vi "Continuous Measurament RT.vi"() -> ()   [LabVIEW 2014]
uses:
  <vilib>/FPGAPlugInAG/sbRIO-9636/niLvFpga_Open_sbRIO-9636.vi
  <vilib>/rvi/interface/common/dynamic/niFpgaDynamicAddResources.vi
  <vilib>/FPGAPlugInAG/Dynamic/niLvFpga_Reset_Dynamic.vi
  <vilib>/FPGAPlugInAG/Dynamic/niLvFpga_Run_Dynamic.vi
  <vilib>/FPGAPlugInAG/Dynamic/niLvFpga_Abort_Dynamic.vi
  <vilib>/FPGAPlugInAG/Dynamic/niLvFpga_Close_Dynamic.vi
  <vilib>/rvi/interface/nirviOpenFPGA/nirviOpenFPGA.xnode
  FPGA Bitfiles/FinalProjectLase_FPGATarget_ContinuousMeasur_qAypivenTJk.lvbitx
  FPGA/Continuous Measurement.vi
  <vilib>/rvi/interface/nirviMethod/nirviMethod.xnode
  <vilib>/rvi/interface/nirviCloseFPGA/nirviCloseFPGA.xnode
  <vilib>/Analysis/NI_AALBase.lvlib
panel:
  in  "Tab Control":T1(tab)
  in  "#Signals":u32(slide)=5 scale=1.0..5.0
  in  "Uncompensated":bool
  in  "Enable triangular scaling":bool=TRUE
  in  "Multiply Factor":dbl[](array[numeric])=[1.0, 0.8, 0.95, 0.85, 0.9]
  in  "Window function":enum16{"None", "Hanning"}(ring)=enum."Hanning"
  in  "Initial Latency points":u32(slide)=260 scale=0.0..1250.0
  in  "lower limit 1":u32(slide)=113 scale=0.0..113.0
  in  "lower limit 2":u32(slide)=738 scale=625.0..738.0
  in  "First FFT bin":i32=5
  in  "Last FFT bin":i32=255
  in  "Extraction Type":T2(ring)=enum."LowPass"
  in  "Low cutoff frequency":dbl=1000000.0 format="%#_13g"
  in  "Poly Grade":dbl=5.0
  in  "side points":i32=6
  in  "polynomial order":i32=3
  out "Distance (m)":dbl format="%0.7f"
  out "Relative Standard Deviation":dbl format="%0.7f"
  in  "Mean distance":i32=1
  out "Measure cycle time":u32
  out "Measurement Uncertainty (m)":dbl format="%0.5f"
  out "Measure Frequency":dbl
  out "Distance (m) Plot":dbl(graph)
  out "Velocity (m/s)":dbl
  out "Velocity (m/s) Plot":dbl(graph)
  in  "STOP":bool
  # "Modulation signal"
  # "Window function"
  # "Residual Extraction"
  # "FFT Parameters"
  # "Low pass filter"
  # "Compensated"
  # "Poly fitting"
  # "SavGolay filter"
  # "Performance"
  # "KHz"
  # "ms"
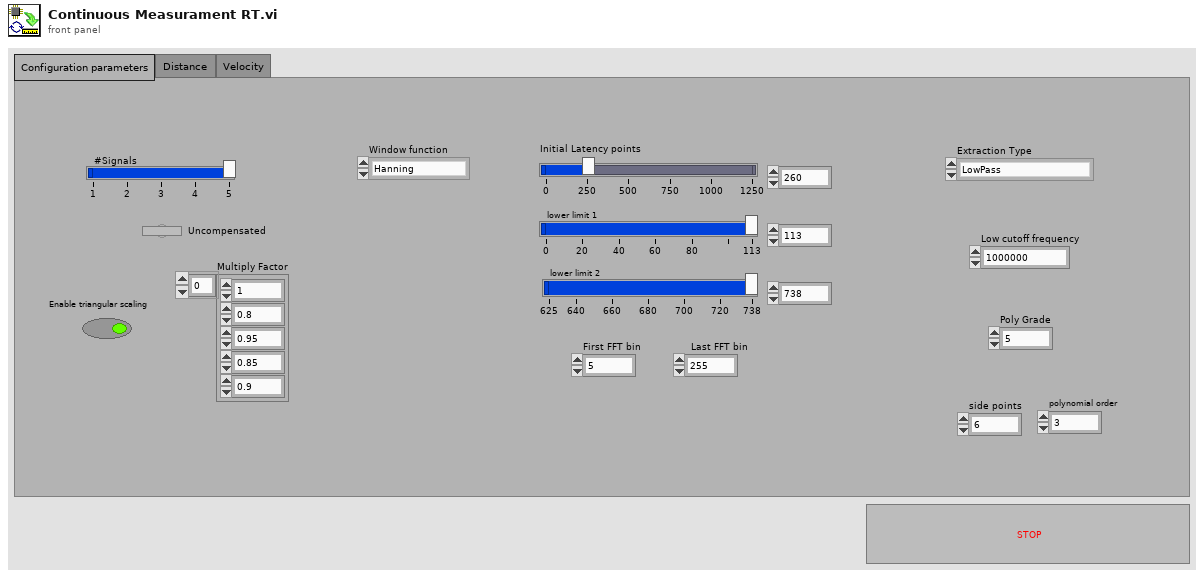
[diagram p1: front panel]
types:
  T1 = enum32{"Configuration parameters", "Distance ", "Velocity"}
  T2 = enum16{"NoSubtract", "StartingCurve", "LowPass", "PolyFitting", "SavGolay"}
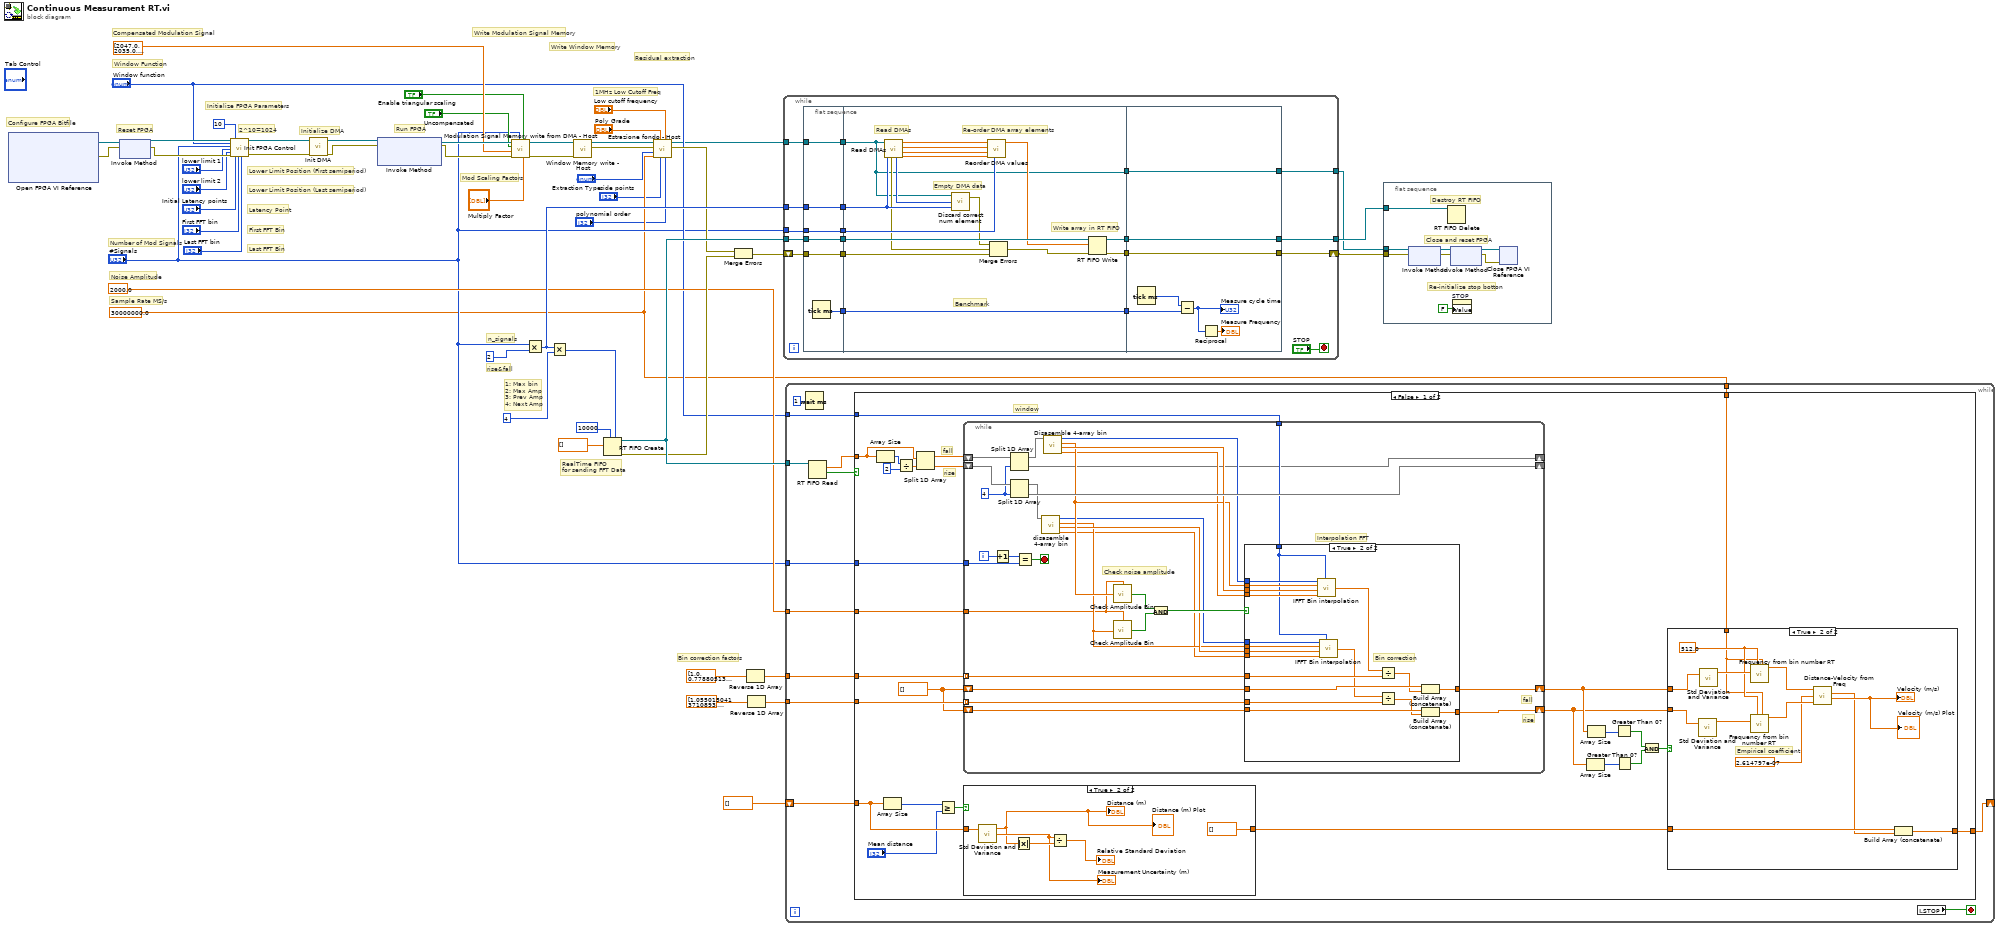
[diagram p0: block diagram]
diagram:
  w10 = 30000000.0
  # "2^10=1024"
  # "Bin correction factors"
  # "Write Modulation Signal Memory"
  # "Residual extraction"
  # "Write Window Memory"
  # "Mod Scaling Factors"
  # "Window Function"
  # "Lower Limit Position (Last semiperiod)"
  # "Lower Limit Position (First semiperiod)"
  # "Latency Point"
  # "Last FFT Bin"
  # "First FFT Bin"
  # "Number of Mod Signals"
  # "Configure FPGA Bitfile"
  # "Run FPGA"
  # "Reset FPGA"
  # "Initialize FPGA Parameters"
  # "Initialize DMA"
  # "1MHz Low Cutoff Freq"
  # "Compensated Modulation Signal"
  # "Sample Rate MS/s"
  # "Noise Amplitude"
  # "n_signals"
  # "rise&fall"
  # "1: Max bin\n2: Max Amp\n3: Prev Amp\n4: Next Amp"
  # "RealTime FIFO \nfor sending FFT Data"
  n1 = xnode "Open FPGA VI Reference"() -> ("FPGA VI Reference Out"=w21:refnum<k20>, "error out"=w20:errorcluster)  [unwired: 2 in]
  n2 = xnode "Invoke Method"("FPGA VI Reference In"=w21, "error in"=w20) -> ("FPGA VI Reference Out"=w18:refnum<k20>, "error out"=w19:errorcluster)
  n3 = call "Init FPGA Control.vi"("FPGA VI Reference In"=w18, "Window Function"="Window function", "n"="#Signals", "lower limit 1"="lower limit 1", "lower limit 2"="lower limit 2", "error in"=w19, "n-bit (2^(nbit) signals for Residual Extraction)"=10, "Initial Latency points"="Initial Latency points", "first FFT bin"="First FFT bin", "last FFT bin"="Last FFT bin") -> ("FPGA VI Reference Out"=w23:refnum<k20>, "error out"=w22:errorcluster)  [unwired: 8 in]
  n4 = call "Init DMA.vi"("error in"=w22, "FPGA VI Reference In"=w23) -> ("error out"=w24:errorcluster, "FPGA VI Reference Out"=w25:refnum<k20>)  [unwired: 8 in]
  n5 = xnode "Invoke Method"("FPGA VI Reference In"=w25, "error in"=w24) -> ("FPGA VI Reference Out"=w38:refnum<k20>, "error out"=w34:errorcluster)  [unwired: 1 in]
  n6 = call "Modulation Signal Memory write from DMA - Host.vi"("Triangular Multiply Factor"="Multiply Factor", "Enable triangular scaling"="Enable triangular scaling", "n"="#Signals", "error in"=w34, "Custom Triangular Signal (fal-ris)"=dbl[] [2047.0, 2035.0, 2022.0, 2010.0, 1997.0, 1985.0, 1972.0, 1960.0, 1948.0, 1935.0, 1923.0, 1911.0, 1899.0, 1886.0, 1874.0, 1862.0, 1850.0, 1838.0, 1825.0, 1813.0, 1801.0, 1789.0, 1777.0, 1765.0, 1753.0, 1741.0, 1729.0, 1717.0, 1705.0, 1693.0, 1681.0, 1669.0, 1657.0, 1645.0, 1634.0, 1622.0, 1610.0, 1598.0, 1586.0, 1575.0, 1563.0, 1551.0, 1540.0, 1528.0, 1516.0, 1505.0, 1493.0, 1481.0, 1470.0, 1458.0, 1447.0, 1435.0, 1424.0, 1412.0, 1401.0, 1389.0, 1378.0, 1366.0, 1355.0, 1344.0, 1332.0, 1321.0, 1310.0, 1298.0, 1287.0, 1276.0, 1265.0, 1253.0, 1242.0, 1231.0, 1220.0, 1209.0, 1198.0, 1186.0, 1175.0, 1164.0, 1153.0, 1142.0, 1131.0, 1120.0, 1109.0, 1098.0, 1087.0, 1076.0, 1065.0, 1055.0, 1044.0, 1033.0, 1022.0, 1011.0, 1000.0, 990.0, 979.0, 968.0, 958.0, 947.0, 936.0, 926.0, 915.0, 904.0, 894.0, 883.0, 873.0, 862.0, 852.0, 841.0, 831.0, 820.0, 810.0, 799.0, 789.0, 778.0, 768.0, 758.0, 747.0, 738.0, 727.0, 719.0, 712.0, 706.0, 700.0, 693.0, 687.0, 680.0, 674.0, 668.0, 661.0, 655.0, 648.0, 642.0, 636.0, 629.0, 623.0, 617.0, 610.0, 604.0, 598.0, 591.0, 584.0, 577.0, 569.0, 560.0, 552.0, 545.0, 538.0, 531.0, 525.0, 519.0, 512.0, 506.0, 500.0, 494.0, 488.0, 482.0, 476.0, 470.0, 464.0, 458.0, 452.0, 446.0, 436.0, 430.0, 424.0, 418.0, 412.0, 406.0, 400.0, 394.0, 388.0, 382.0, 376.0, 370.0, 364.0, 358.0, 352.0, 346.0, 338.0, 332.0, 325.0, 319.0, 313.0, 307.0, 301.0, 295.0, 290.0, 284.0, 278.0, 272.0, 267.0, 261.0, 255.0, 249.0, 244.0, 238.0, 232.0, 227.0, 221.0, 215.0, 209.0, 204.0, 198.0, 192.0, 187.0, 181.0, 175.0, 170.0, 164.0, 158.0, 153.0, 147.0, 141.0, 136.0, 130.0, 124.0, 119.0, 113.0, 108.0, 102.0, 96.0, 91.0, 85.0, 79.0, 74.0, 68.0, 62.0, 57.0, 51.0, 45.0, 39.0, 34.0, 28.0, 22.0, 16.0, 11.0, 5.0, 0.0, -6.0, -11.0, -17.0, -22.0, -28.0, -33.0, -39.0, -44.0, -50.0, -55.0, -61.0, -66.0, -72.0, -77.0, -83.0, -88.0, -94.0, -99.0, -105.0, -110.0, -116.0, -121.0, -127.0, -132.0, -137.0, -143.0, -148.0, -154.0, -159.0, -165.0, -170.0, -176.0, -181.0, -186.0, -192.0, -197.0, -203.0, -208.0, -214.0, -219.0, -224.0, -230.0, -235.0, -241.0, -246.0, -251.0, -257.0, -262.0, -268.0, -273.0, -278.0, -284.0, -289.0, -295.0, -300.0, -305.0, -311.0, -316.0, -321.0, -327.0, -332.0, -337.0, -343.0, -348.0, -354.0, -359.0, -364.0, -370.0, -375.0, -380.0, -386.0, -391.0, -397.0, -402.0, -407.0, -413.0, -418.0, -423.0, -429.0, -434.0, -439.0, -445.0, -450.0, -455.0, -461.0, -466.0, -471.0, -477.0, -482.0, -487.0, -493.0, -498.0, -503.0, -509.0, -514.0, -519.0, -525.0, -530.0, -535.0, -540.0, -546.0, -551.0, -556.0, -562.0, -567.0, -572.0, -578.0, -583.0, -588.0, -593.0, -599.0, -604.0, -609.0, -615.0, -620.0, -625.0, -630.0, -636.0, -641.0, -646.0, -651.0, -657.0, -662.0, -667.0, -673.0, -678.0, -683.0, -688.0, -694.0, -699.0, -704.0, -709.0, -715.0, -720.0, -725.0, -730.0, -736.0, -741.0, -746.0, -751.0, -757.0, -762.0, -767.0, -772.0, -778.0, -783.0, -788.0, -793.0, -799.0, -804.0, -809.0, -814.0, -820.0, -825.0, -830.0, -835.0, -841.0, -846.0, -851.0, -856.0, -862.0, -867.0, -872.0, -877.0, -883.0, -888.0, -893.0, -898.0, -903.0, -909.0, -914.0, -919.0, -924.0, -930.0, -935.0, -940.0, -945.0, -951.0, -956.0, -961.0, -966.0, -971.0, -977.0, -982.0, -987.0, -992.0, -998.0, -1003.0, -1008.0, -1013.0, -1018.0, -1024.0, -1029.0, -1034.0, -1039.0, -1045.0, -1050.0, -1055.0, -1060.0, -1065.0, -1071.0, -1076.0, -1081.0, -1086.0, -1092.0, -1097.0, -1102.0, -1107.0, -1112.0, -1118.0, -1123.0, -1128.0, -1133.0, -1138.0, -1144.0, -1149.0, -1154.0, -1159.0, -1165.0, -1170.0, -1175.0, -1180.0, -1185.0, -1191.0, -1196.0, -1201.0, -1206.0, -1211.0, -1217.0, -1222.0, -1227.0, -1232.0, -1237.0, -1243.0, -1248.0, -1253.0, -1258.0, -1263.0, -1269.0, -1274.0, -1279.0, -1284.0, -1289.0, -1295.0, -1300.0, -1305.0, -1310.0, -1315.0, -1321.0, -1326.0, -1331.0, -1336.0, -1341.0, -1347.0, -1352.0, -1357.0, -1362.0, -1367.0, -1373.0, -1378.0, -1383.0, -1388.0, -1393.0, -1399.0, -1404.0, -1409.0, -1414.0, -1419.0, -1425.0, -1430.0, -1435.0, -1440.0, -1445.0, -1450.0, -1456.0, -1461.0, -1466.0, -1471.0, -1476.0, -1482.0, -1487.0, -1492.0, -1497.0, -1502.0, -1508.0, -1513.0, -1518.0, -1523.0, -1528.0, -1534.0, -1539.0, -1544.0, -1549.0, -1554.0, -1560.0, -1565.0, -1570.0, -1575.0, -1580.0, -1586.0, -1591.0, -1596.0, -1601.0, -1606.0, -1612.0, -1617.0, -1622.0, -1627.0, -1632.0, -1637.0, -1643.0, -1648.0, -1653.0, -1658.0, -1663.0, -1669.0, -1674.0, -1679.0, -1684.0, -1689.0, -1695.0, -1700.0, -1705.0, -1710.0, -1715.0, -1721.0, -1726.0, -1731.0, -1736.0, -1741.0, -1747.0, -1752.0, -1757.0, -1762.0, -1767.0, -1773.0, -1778.0, -1783.0, -1788.0, -1793.0, -1799.0, -1804.0, -1809.0, -1814.0, -1819.0, -1825.0, -1830.0, -1835.0, -1840.0, -1845.0, -1851.0, -1856.0, -1861.0, -1866.0, -1871.0, -1876.0, -1882.0, -1887.0, -1892.0, -1897.0, -1902.0, -1908.0, -1913.0, -1918.0, -1923.0, -1928.0, -1934.0, -1939.0, -1944.0, -1949.0, -1954.0, -1960.0, -1965.0, -1970.0, -1975.0, -1980.0, -1986.0, -1991.0, -1996.0, -2001.0, -2006.0, -2012.0, -2017.0, -2022.0, -2027.0, -2032.0, -2038.0, -2043.0, -2048.0, -2047.0, -2037.0, -2027.0, -2017.0, -2007.0, -1997.0, -1987.0, -1977.0, -1967.0, -1957.0, -1947.0, -1937.0, -1927.0, -1917.0, -1907.0, -1897.0, -1888.0, -1878.0, -1868.0, -1858.0, -1848.0, -1838.0, -1828.0, -1819.0, -1809.0, -1799.0, -1789.0, -1780.0, -1770.0, -1760.0, -1750.0, -1741.0, -1731.0, -1721.0, -1712.0, -1702.0, -1692.0, -1683.0, -1673.0, -1663.0, -1654.0, -1644.0, -1635.0, -1625.0, -1615.0, -1606.0, -1596.0, -1587.0, -1577.0, -1568.0, -1558.0, -1549.0, -1539.0, -1530.0, -1520.0, -1511.0, -1501.0, -1492.0, -1483.0, -1473.0, -1464.0, -1454.0, -1445.0, -1436.0, -1426.0, -1417.0, -1408.0, -1398.0, -1389.0, -1380.0, -1371.0, -1361.0, -1352.0, -1343.0, -1334.0, -1324.0, -1315.0, -1306.0, -1297.0, -1288.0, -1278.0, -1269.0, -1260.0, -1251.0, -1242.0, -1233.0, -1224.0, -1215.0, -1205.0, -1196.0, -1187.0, -1178.0, -1169.0, -1160.0, -1151.0, -1142.0, -1133.0, -1124.0, -1115.0, -1106.0, -1097.0, -1088.0, -1080.0, -1071.0, -1062.0, -1053.0, -1044.0, -1035.0, -1026.0, -1017.0, -1009.0, -1000.0, -991.0, -982.0, -973.0, -965.0, -953.0, -944.0, -935.0, -920.0, -906.0, -889.0, -871.0, -854.0, -842.0, -834.0, -826.0, -818.0, -810.0, -802.0, -794.0, -786.0, -778.0, -770.0, -762.0, -754.0, -746.0, -739.0, -731.0, -723.0, -715.0, -707.0, -699.0, -690.0, -682.0, -672.0, -661.0, -651.0, -639.0, -627.0, -616.0, -606.0, -598.0, -591.0, -584.0, -577.0, -570.0, -563.0, -556.0, -549.0, -542.0, -535.0, -528.0, -520.0, -513.0, -506.0, -499.0, -492.0, -485.0, -478.0, -471.0, -464.0, -457.0, -451.0, -444.0, -437.0, -430.0, -423.0, -416.0, -409.0, -400.0, -390.0, -382.0, -373.0, -364.0, -356.0, -349.0, -343.0, -336.0, -330.0, -323.0, -317.0, -310.0, -304.0, -297.0, -291.0, -284.0, -278.0, -271.0, -265.0, -258.0, -252.0, -245.0, -239.0, -232.0, -226.0, -219.0, -213.0, -207.0, -200.0, -194.0, -187.0, -181.0, -175.0, -168.0, -162.0, -156.0, -149.0, -143.0, -136.0, -128.0, -121.0, -114.0, -107.0, -100.0, -93.0, -87.0, -80.0, -74.0, -68.0, -62.0, -56.0, -50.0, -44.0, -38.0, -32.0, -26.0, -20.0, -14.0, -8.0, -2.0, 5.0, 11.0, 17.0, 23.0, 29.0, 35.0, 41.0, 47.0, 53.0, 59.0, 65.0, 70.0, 76.0, 82.0, 88.0, 94.0, 100.0, 106.0, 112.0, 118.0, 124.0, 130.0, 136.0, 142.0, 148.0, 154.0, 161.0, 167.0, 174.0, 180.0, 186.0, 192.0, 198.0, 204.0, 210.0, 215.0, 221.0, 227.0, 233.0, 238.0, 244.0, 250.0, 255.0, 261.0, 267.0, 273.0, 278.0, 284.0, 290.0, 295.0, 301.0, 307.0, 312.0, 318.0, 324.0, 329.0, 335.0, 341.0, 346.0, 352.0, 358.0, 363.0, 369.0, 374.0, 380.0, 386.0, 391.0, 397.0, 402.0, 408.0, 414.0, 419.0, 425.0, 430.0, 436.0, 441.0, 447.0, 453.0, 458.0, 464.0, 470.0, 475.0, 481.0, 487.0, 493.0, 499.0, 504.0, 510.0, 516.0, 521.0, 527.0, 532.0, 538.0, 543.0, 549.0, 554.0, 560.0, 565.0, 571.0, 576.0, 582.0, 587.0, 593.0, 598.0, 604.0, 609.0, 614.0, 620.0, 625.0, 631.0, 636.0, 642.0, 647.0, 653.0, 658.0, 663.0, 669.0, 674.0, 680.0, 685.0, 691.0, 696.0, 701.0, 707.0, 712.0, 718.0, 723.0, 728.0, 734.0, 739.0, 745.0, 750.0, 755.0, 761.0, 766.0, 772.0, 777.0, 782.0, 788.0, 793.0, 798.0, 804.0, 809.0, 815.0, 820.0, 826.0, 831.0, 837.0, 842.0, 847.0, 853.0, 858.0, 863.0, 869.0, 874.0, 880.0, 885.0, 890.0, 895.0, 901.0, 906.0, 911.0, 917.0, 922.0, 927.0, 933.0, 938.0, 943.0, 948.0, 954.0, 959.0, 964.0, 970.0, 975.0, 980.0, 985.0, 991.0, 996.0, 1001.0, 1006.0, 1012.0, 1017.0, 1022.0, 1027.0, 1033.0, 1038.0, 1043.0, 1048.0, 1054.0, 1059.0, 1064.0, 1069.0, 1075.0, 1080.0, 1085.0, 1090.0, 1096.0, 1101.0, 1106.0, 1111.0, 1116.0, 1122.0, 1127.0, 1132.0, 1137.0, 1143.0, 1148.0, 1153.0, 1158.0, 1163.0, 1169.0, 1174.0, 1179.0, 1184.0, 1190.0, 1195.0, 1200.0, 1205.0, 1211.0, 1216.0, 1221.0, 1226.0, 1231.0, 1237.0, 1242.0, 1247.0, 1252.0, 1257.0, 1262.0, 1268.0, 1273.0, 1278.0, 1283.0, 1288.0, 1293.0, 1298.0, 1304.0, 1309.0, 1314.0, 1319.0, 1324.0, 1329.0, 1334.0, 1340.0, 1345.0, 1350.0, 1355.0, 1360.0, 1365.0, 1370.0, 1375.0, 1381.0, 1386.0, 1391.0, 1396.0, 1401.0, 1406.0, 1411.0, 1416.0, 1421.0, 1427.0, 1432.0, 1437.0, 1442.0, 1447.0, 1452.0, 1457.0, 1462.0, 1467.0, 1472.0, 1478.0, 1483.0, 1488.0, 1493.0, 1498.0, 1503.0, 1508.0, 1513.0, 1518.0, 1523.0, 1528.0, 1534.0, 1539.0, 1544.0, 1549.0, 1554.0, 1559.0, 1564.0, 1569.0, 1574.0, 1579.0, 1584.0, 1589.0, 1595.0, 1600.0, 1605.0, 1610.0, 1615.0, 1620.0, 1625.0, 1630.0, 1635.0, 1640.0, 1645.0, 1650.0, 1655.0, 1660.0, 1666.0, 1671.0, 1676.0, 1681.0, 1686.0, 1691.0, 1696.0, 1701.0, 1706.0, 1711.0, 1716.0, 1721.0, 1726.0, 1731.0, 1736.0, 1741.0, 1746.0, 1751.0, 1757.0, 1762.0, 1767.0, 1772.0, 1777.0, 1782.0, 1787.0, 1792.0, 1797.0, 1802.0, 1807.0, 1812.0, 1817.0, 1822.0, 1827.0, 1832.0, 1837.0, 1842.0, 1847.0, 1852.0, 1857.0, 1862.0, 1867.0, 1872.0, 1877.0, 1883.0, 1888.0, 1893.0, 1898.0, 1903.0, 1908.0, 1913.0, 1918.0, 1923.0, 1928.0, 1933.0, 1938.0, 1943.0, 1948.0, 1953.0, 1958.0, 1963.0, 1968.0, 1973.0, 1978.0, 1983.0, 1988.0, 1993.0, 1998.0, 2003.0, 2008.0, 2013.0, 2018.0, 2023.0, 2028.0, 2033.0, 2038.0, 2043.0, 2048.0] ("appended array"), "Modulation signal (pendenza dritta)?"="Uncompensated", "FPGA VI Reference In"=w38) -> ("error out"=w31:errorcluster, "FPGA VI Reference Out"=w32:refnum<k20>)  [unwired: 2 in, 1 out]
  n7 = Multiply(x="#Signals", y=u32 2 ("elements in array (1)")) -> (x*y=w47:u32)
  n8 = Multiply(x=w47, y=u32 4 ("elements in array (1)")) -> (x*y=w48:u32)
  n9 = call "Window Memory write - Host.vi"("error in"=w31, "FPGA VI Reference In"=w32) -> ("error out"=w30:errorcluster, "FPGA VI Reference Out"=w29:refnum<k20>)  [unwired: 7 in, 1 out]
  n10 = RT FIFO Create(1:dbl[] [] ("first subarray"), 4:u32 10000 ("size (10)"), 6:w48) -> (8:w51:refnum<k33>, 11:w45:errorcluster)  [unwired: 5 in, 1 out]
  n11 = call "Estrazione fondo - Host.vi"("polynomial order"="polynomial order", "LowPass Filter: Low cutoff frequency"="Low cutoff frequency", "side points"="side points", "PolyFitting: Poly Grade"="Poly Grade", "Low Pass filter: Sampling freq: fs"=w10, "SubtractionType"="Extraction Type", "error in"=w30, "FPGA VI Reference In"=w29) -> ("error out"=w26:errorcluster, "FPGA VI Reference Out"=w9:refnum<k20>)  [unwired: 2 out]
  n12 = Merge Errors(w26, w45) -> (w44:errorcluster)
  n13 = Reverse 1D Array(array=dbl[] [1.0, 0.7788051374952276, 0.9586568902543302, 0.8395566206470091, 0.903068410955916] ("mean factor 1")) -> (reversed array=w41:dbl[])
  n14 = Reverse 1D Array(array=dbl[] [1.0550150413710893, 0.8807744280543515, 1.0096480344577006, 0.9233799836458207, 0.9653106595082892] ("mean factor 2")) -> (reversed array=w39:dbl[])
  n15 = while {
    tunnel: w51 -> [w71]
    tunnel: w47 -> [w65]
    shift-right: [w69] -> w7
    shift-left: w44 -> [w70]
    tunnel: "#Signals" -> [w68]
    tunnel: [w67] -> w8
    tunnel: w9 -> [w56]
    tunnel: [w53] -> w6
    stop <- "STOP" stop-if-true
    n16 = flat-sequence {
      tunnel: w65 -> [w74]
      tunnel: w68 -> [w75]
      tunnel: w70 -> [w76]
      tunnel: w71 -> [w77]
      tunnel: [w77] -> w64
      tunnel: [w76] -> w63
      tunnel: [w75] -> w62
      tunnel: [w74] -> w61
      tunnel: [w73] -> w60
      tunnel: w56 -> [w72]
      tunnel: [w72] -> w55
      tunnel: w64 -> [w94]
      tunnel: w63 -> [w80]
      tunnel: w62 -> [w86]
      tunnel: w61 -> [w83]
      tunnel: w60 -> [w91]
      tunnel: [w93] -> w59
      tunnel: [w92] -> w58
      tunnel: [w91] -> w57
      tunnel: w55 -> [w78]
      tunnel: [w78] -> w54
      tunnel: [w100] -> w67
      tunnel: [w101] -> w69
      tunnel: w59 -> [w101]
      tunnel: w58 -> [w100]
      tunnel: w57 -> [w99]
      tunnel: w54 -> [w95]
      tunnel: [w95] -> w53
      frame #0 {
        n17 = Tick Count (ms)() -> (millisecond timer value=w73:u32)
      }
      frame #1 {
        # "Benchmark"
        # "Write array in RT FIFO"
        # "Re-order DMA array elements"
        # "Empty DMA data"
        # "Read DMAs"
        n18 = call "Read DMAs.vi"("Number of Elements"=w83, "FPGA VI Reference In"=w78) -> ("Next Amp"=w87:dbl[], "Prev Amp"=w88:dbl[], "Max Amp"=w89:dbl[], "Max bin"=w90:dbl[], "Elements Remaining in Max bin DMA"=w84:u32, "error out"=w81:errorcluster)  [unwired: 4 in]
        n19 = call "Discard correct num element.vi"("Read packet dim"=w83, "Element Remaing in Queue"=w84, "FPGA VI Reference In"=w78) -> ("error out"=w82:errorcluster)  [unwired: 1 in]
        n20 = call "Reorder DMA values.vi"("Number of signals"=w86, "Next Amp array"=w87, "Prev Amp array"=w88, "Max Amp array"=w89, "Max bin array"=w90) -> ("Ordered array"=w85:dbl[])  [unwired: 6 in]
        n21 = Merge Errors(w82, w81, w80) -> (w79:errorcluster)
        n22 = RT FIFO Write(0:w94, 1:w85, 3:w79) -> (8:w92:refnum<k33>, 11:w93:errorcluster)  [unwired: 2 in, 2 out]
      }
      frame #2 {
        n23 = Tick Count (ms)() -> (millisecond timer value=w98:u32)
        n24 = Subtract(x=w98, y=w99) -> (x-y=w97:u32)
        "Measure cycle time" <- w97
        n25 = Reciprocal(x=w97) -> (1/x=→"Measure Frequency":dbl)
      }
    }
  }
  n26 = while {
    tunnel: w51 -> [w114]
    tunnel: "Window function" -> [w111]
    tunnel: "#Signals" -> [w110]
    shift-right: [w102] -> _
    shift-left: dbl[] [] ("appended array") -> [w109]
    tunnel: w10 -> [w108]
    tunnel: w41 -> [w107]
    tunnel: w39 -> [w106]
    tunnel: 2000.0 ("Threshold Amp") -> [w105]
    stop <- w103 stop-if-true
    n27 = Wait (ms)(milliseconds to wait=u32 1) -> ()  [unwired: 1 out]
    n28 = RT FIFO Read(0:w114) -> (9:w112:dbl[], 10:w113:bool)  [unwired: 3 in, 3 out]
    n29 = case shown="False" w113 {
      tunnel: w112 -> [w140 _]
      tunnel: w111 -> [w139 _]
      tunnel: w110 -> [w137 _]
      tunnel: w109 -> [w133 w213]
      tunnel: [w131 w213] -> w102
      tunnel: w108 -> [w122 _]
      tunnel: w107 -> [w130 _]
      tunnel: w106 -> [w129 _]
      tunnel: w105 -> [w128 _]
      frame False {
        w120 = dbl[] [] ("appended array")
        # "window"
        # "rise"
        # "fall"
        n30 = Array Size(array=w140) -> (size(s)=w127:i32)
        n31 = Array Size(array=w133) -> (size(s)=w134:i32)
        n32 = Divide(x=w127, y=2) -> (x/y=w125:dbl)
        n33 = Split 1D Array(array=w140, index=w125) -> (first subarray=w121:dbl[], second subarray=w138:dbl[])
        n34 = Greater Or Equal?(x=w134, y="Mean distance") -> (x >= y?=w124:bool)
        n35 = while {
          shift-right: [w163] -> _
          shift-left: w121 -> [w191]
          shift-right: [w184] -> _
          shift-left: w138 -> [w190]
          tunnel: w139 -> [w180]
          tunnel: w137 -> [w188]
          shift-right: [w179] -> w136
          shift-left: w120 -> [w177]
          shift-right: [w178] -> w118
          shift-left: w120 -> [w176]
          tunnel: w130 -> [w175] mode=indexing
          tunnel: w129 -> [w174] mode=indexing
          tunnel: w128 -> [w162]
          i -> [w185]
          stop <- w189 stop-if-true
          w187 = 4 ("x")
          # "Interpolation FFT"
          # "Check noise amplitude"
          # "rise"
          # "fall"
          n36 = Increment(x=w185) -> (x+1=w186:i32)
          n37 = Split 1D Array(array=w191, index=w187) -> (first subarray=w173:dbl[], second subarray=w163:dbl[])
          n38 = Split 1D Array(array=w190, index=w187) -> (first subarray=w172:dbl[], second subarray=w184:dbl[])
          n39 = Equal?(x=w186, y=w188) -> (x = y?=w189:bool)
          n40 = call "disasemble 4-array bin.vi"("4-Array Bin-Amp"=w172) -> ("Next Amp"=w165:dbl, "Prev amp"=w167:dbl, "Max amp"=w166:dbl, "Max bin"=w168:i32)  [unwired: 7 in]
          n41 = call "Disasemble 4-array bin.vi"("4-Array Bin-Amp"=w173) -> ("Next Amp"=w169:dbl, "Prev amp"=w171:dbl, "Max amp"=w170:dbl, "Max bin"=w164:i32)  [unwired: 7 in]
          n42 = call "Check Amplitude Bin.vi"("Threshold Amp"=w162, "Max Amp"=w170) -> ("Check Amp Ok?"=w183:bool)  [unwired: 2 in]
          n43 = call "Check Amplitude Bin.vi"("Threshold Amp"=w162, "Max Amp"=w166) -> ("Check Amp Ok?"=w182:bool)  [unwired: 2 in]
          n44 = And(x=w183, y=w182) -> (x .and. y?=w181:bool)
          n45 = case shown="True" w181 {
            tunnel: w167 -> [_ w212]
            tunnel: w165 -> [_ w211]
            tunnel: w166 -> [_ w210]
            tunnel: w168 -> [_ w209]
            tunnel: w164 -> [_ w208]
            tunnel: w171 -> [_ w207]
            tunnel: w170 -> [_ w206]
            tunnel: w169 -> [_ w205]
            tunnel: w180 -> [_ w204]
            tunnel: [w193 w199] -> w179
            tunnel: [w192 w198] -> w178
            tunnel: w177 -> [w193 w203]
            tunnel: w176 -> [w192 w202]
            tunnel: w175 -> [_ w201]
            tunnel: w174 -> [_ w200]
            frame False {
            }
            frame True {
              # "Bin correction"
              n46 = call "IFFT Bin interpolation.vi"("Max Bin"=w208, "Max Amp"=w206, "Prev Amp"=w207, "Next Amp"=w205, "Windowing"=w204) -> ("Interpolate Bin"=w197:dbl)
              n47 = call "IFFT Bin interpolation.vi"("Max Bin"=w209, "Max Amp"=w210, "Prev Amp"=w212, "Next Amp"=w211, "Windowing"=w204) -> ("Interpolate Bin"=w196:dbl)
              n48 = Divide(x=w197, y=w201) -> (x/y=w195:dbl)
              n49 = Divide(x=w196, y=w200) -> (x/y=w194:dbl)
              n50 = Build Array (concatenate)(w203, w195) -> (w199:dbl[])
              n51 = Build Array (concatenate)(w202, w194) -> (w198:dbl[])
            }
          }
        }
        n52 = case shown="True" w124 {
          tunnel: w133 -> [w141 w146]
          tunnel: [w141 dbl[] [] ("appended array")] -> w132
          frame False {
          }
          frame True {
            n53 = call <vilib>:"Std Deviation and Variance.vi"("X"=w146) -> ("mean"=w142:dbl, "standard deviation"=w144:dbl)  [unwired: 1 in, 1 out]
            "Distance (m)" <- w142
            "Distance (m) Plot" <- w142
            "Measurement Uncertainty (m)" <- w144
            n54 = Absolute Value(x=w142) -> (abs(x)=w147:dbl)
            n55 = Divide(x=w144, y=w147) -> (x/y=→"Relative Standard Deviation":dbl)
          }
        }
        n56 = Array Size(array=w118) -> (size(s)=w119:i32)
        n57 = Array Size(array=w136) -> (size(s)=w135:i32)
        n58 = Greater Than 0?(x=w135) -> (x > 0?=w115:bool)
        n59 = Greater Than 0?(x=w119) -> (x > 0?=w116:bool)
        n60 = And(x=w115, y=w116) -> (x .and. y?=w117:bool)
        n61 = case shown="True" w117 {
          tunnel: w136 -> [_ w161]
          tunnel: w118 -> [_ w160]
          tunnel: w132 -> [w148 w159]
          tunnel: [w148 w158] -> w131
          tunnel: w122 -> [_ w154]
          frame False {
          }
          frame True {
            w155 = 512.0 ("FFT size")
            # "Empirical coefficient"
            n62 = call <vilib>:"Std Deviation and Variance.vi"("X"=w160) -> ("mean"=w156:dbl)  [unwired: 1 in, 2 out]
            n63 = call <vilib>:"Std Deviation and Variance.vi"("X"=w161) -> ("mean"=w157:dbl)  [unwired: 1 in, 2 out]
            n64 = call "Frequency from bin number RT.vi"("Sample Rate (S/s)"=w154, "FFT size"=w155, "Bin number"=w157) -> ("Detected Frequency (Hz)"=w153:dbl)  [unwired: 8 in]
            n65 = call "Frequency from bin number RT.vi"("Sample Rate (S/s)"=w154, "FFT size"=w155, "Bin number"=w156) -> ("Detected Frequency (Hz)"=w152:dbl)  [unwired: 8 in]
            n66 = call "Distance-Velocity from Freq.vi"("freq_falling"=w153, "Empirical Distance Costant"=2.614797e-07, "freq_rising"=w152) -> ("Distance (m)"=w149:dbl, "Velocity (m/s)"=→"Velocity (m/s)" →"Velocity (m/s) Plot":dbl)  [unwired: 2 in, 2 out]
            n67 = Build Array (concatenate)(w159, w149) -> (w158:dbl[])
          }
        }
      }
      frame True {
      }
    }
    n68 = local read "STOP"() -> (w103:bool)
  }
  n69 = flat-sequence {
    tunnel: w7 -> [w221]
    tunnel: w8 -> [w215]
    tunnel: w6 -> [w214]
    frame #0 {
      # "Re-initialize stop botton"
      # "Destroy RT FIFO"
      # "Close and reset FPGA"
      n70 = xnode "Invoke Method"("FPGA VI Reference In"=w214, "error in"=w221) -> ("FPGA VI Reference Out"=w218:refnum<k20>, "error out"=w217:errorcluster)
      n71 = RT FIFO Delete(0:w215) -> ()  [unwired: 2 in, 1 out]
      n72 = xnode "Invoke Method"("FPGA VI Reference In"=w218, "error in"=w217) -> ("FPGA VI Reference Out"=w219:refnum<k20>, "error out"=w220:errorcluster)
      n73 = property on="STOP" class="Bool (strict)"("Value"=FALSE ("stop")) -> ()  [unwired: 2 in, 2 out]
      n74 = xnode "Close FPGA VI Reference"("FPGA VI Reference In"=w219, "error in"=w220) -> ()  [unwired: 1 out]
    }
  }
